vi "DataToRead.vi"(8 "error in (no error)":errorcluster, 11 "QueueReader in":refnum<class "QueueReader.lvclass">) -> (0 "error out":errorcluster, 2 "Data available?":bool, 3 "QueueReader out":refnum<class "QueueReader.lvclass">)   [LabVIEW 2025, in "QueueReader.lvclass"]
doc: "Returns TRUE if there is any data to read from the remote host"
uses:
  QueueReader.lvclass
  QueueReader.lvclass/QueueReader.ctl
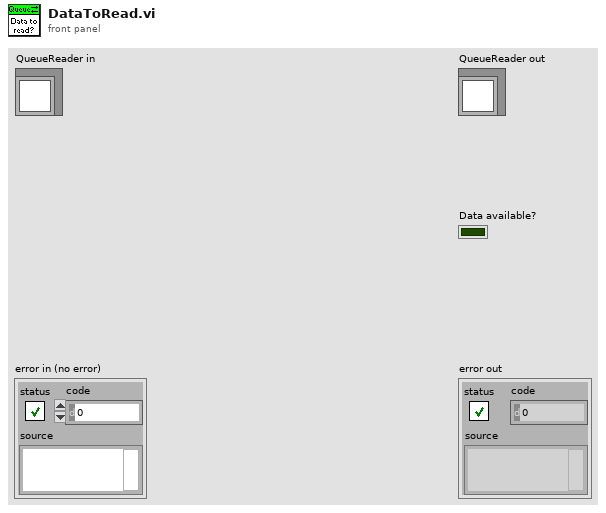
[diagram p1: front panel]
types:
  T1 = typedef "response queue.ctl" = refnum<queue>
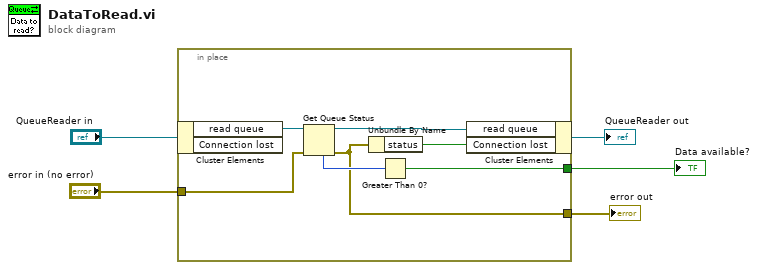
[diagram p0: block diagram]
diagram:
  n1 = in-place "In Place Element Structure" {
    in-place-border: [w9] -> w1
    in-place-border: "error in (no error)" -> [w8]
    in-place-border: [w7] -> w3
    n2 = in-place-cluster #1("QueueReader in") -> ("read queue"=w12:T1)  [unwired: 1 out]
    n3 = Get Queue Status(queue=w12, error in (no error)=w8) -> (queue out=w10:T1, error out=w7:errorcluster, # elements in queue=w11:i32)  [unwired: 1 in, 5 out]
    n4 = Unbundle By Name(w7) -> ("status"=w6:bool)
    n5 = Greater Than 0?(x=w11) -> (x > 0?=w9:bool)
    n6 = in-place-cluster #1("read queue"=w10, "Connection lost"=w6) -> (→"QueueReader out":refnum<class "QueueReader.lvclass">)
  }
  "error out" <- w3
  "Data available?" <- w1
